vi "LVFunction_Imop_Compute_ModalCoef From Slopes.vi"(0 "HasoSlopes.lvclass":refnum<class "HasoSlopes.lvclass">, 5 "ComputePhaseSet.lvclass":refnum<class "ComputePhaseSet.lvclass">, 7 "ModalCoef.lvclass":refnum<class "ModalCoef.lvclass">, 11 "error constant":errorcluster) -> (6 "ComputePhaseSet.lvclass (dup)":refnum<class "ComputePhaseSet.lvclass">, 8 "ModalCoef.lvclass (dup)":refnum<class "ModalCoef.lvclass">, 15 "error out":errorcluster)   [LabVIEW 2020]
doc: "Compute modal coefficients that represent slopes in a given basis of\npolynomials provided by ComputePhaseSet.\n\n--------------------------------------------------------------------------------\n\nHasoDataIn\n HasoData object.\n\nHasoDataOut\n HasoData object.\n\nComputePhaseSet\n cComputePhaseSet object.\n\nmodalCoef\n cModalCoef object.\n\nErrorIn\n Error\nErrorOut\n Error"
uses:
  HasoSlopes.lvclass
  ComputePhaseSet.lvclass
  ModalCoef.lvclass
  LVClass_ModalCoef Read ModalCoef.vi
  LVClass_ComputePhaseSet Read ComputePhaseSet.vi
  LVClass_HasoSlopes Read HasoSlopes _ property.vi
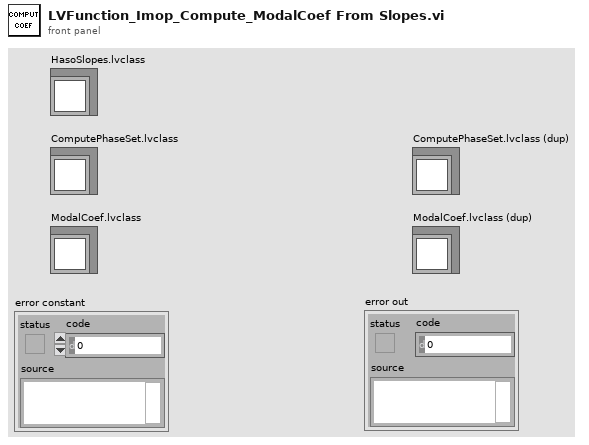
[diagram p1: front panel]
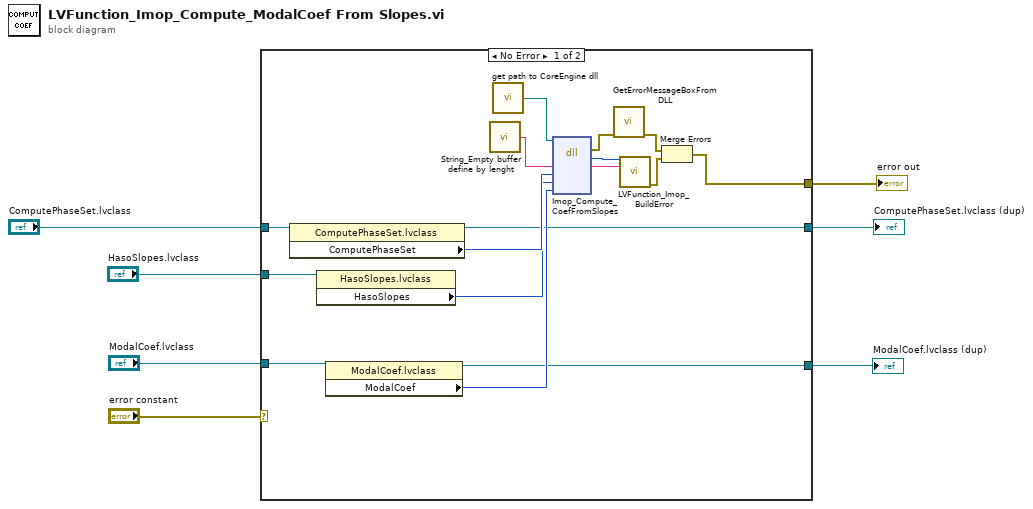
[diagram p0: block diagram]
diagram:
  n1 = case shown="No Error" "error constant" {
    selector: "error constant" -> [_ w26]
    tunnel: "HasoSlopes.lvclass" -> [w18 _]
    tunnel: "ComputePhaseSet.lvclass" -> [w17 w25]
    tunnel: [w10 w26] -> w6
    tunnel: "ModalCoef.lvclass" -> [w14 w24]
    tunnel: [w9 w24] -> w2
    tunnel: [w8 w25] -> w1
    frame No Error {
      n2 = property class="ComputePhaseSet.lvclass"(reference=w17) -> (reference out=w8:refnum<class "ComputePhaseSet.lvclass">, "ComputePhaseSet"=w16:i32)  [unwired: 1 in, 1 out]
      n3 = property class="HasoSlopes.lvclass"(reference=w18) -> ("HasoSlopes"=w15:i32)  [unwired: 1 in, 2 out]
      n4 = property class="ModalCoef.lvclass"(reference=w14) -> (reference out=w9:refnum<class "ModalCoef.lvclass">, "ModalCoef"=w13:u32)  [unwired: 1 in, 1 out]
      n5 = call "String_Empty buffer define by lenght.vi"() -> ("Empty buffer"=w21:string)  [unwired: 1 in]
      n6 = call "get path to CoreEngine dll.vi"() -> ("path to c_interface_vc100.dll"=w20:path)  [unwired: 12 in, 3 out]
      n7 = dll-call lib="D:/FLE/0.Code/CoreEngine4_Suite/LV2011_interface/DLLs/c_interface_vc100.dll" fn="Imop_Compute_CoefFromSlopes"(path in=w20, "message"=w21, "ComputePhaseSet"=w16, "HasoSlopes"=w15, "ModalCoeffs"=w13) -> (error out=w19:errorcluster, "return type"=w23:i32, "message"=w22:string)  [unwired: 5 in, 1 out]
      n8 = call "GetErrorMessageBoxFromDLL.vi"("error IN"=w19) -> ("error OUT"=w12:errorcluster)  [unwired: 10 in]
      n9 = call "LVFunction_Imop_BuildError.vi"("code"=w23, "String to Prepend to source (\"\")"=w22) -> ("error out"=w11:errorcluster)  [unwired: 13 in]
      n10 = Merge Errors(w12, w11) -> (w10:errorcluster)
    }
    frame Error {
    }
  }
  "error out" <- w6
  "ModalCoef.lvclass (dup)" <- w2
  "ComputePhaseSet.lvclass (dup)" <- w1
